vi "Read Landmarks From Text File.vi"(8 "error in":errorcluster, 10 "root VI's Path":path, 11 "File Name":string) -> (0 "error out":errorcluster, 3 "Landmarks":cluster{dbl, dbl}[](array[cluster]))   [LabVIEW 2009]
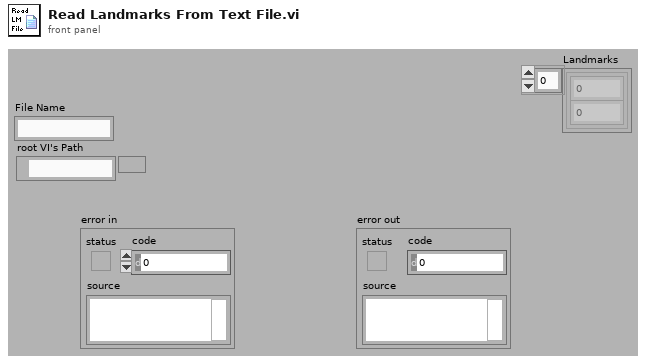
[diagram p1: front panel]
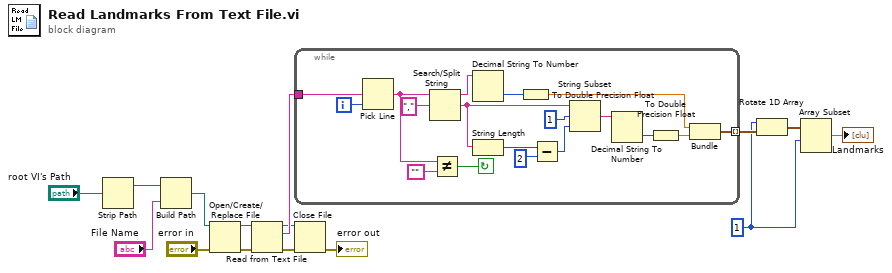
[diagram p0: block diagram]
diagram:
  w6 = 1 ("n")
  n1 = Strip Path(path="root VI's Path") -> (stripped path=w3:path)  [unwired: 1 out]
  n2 = Build Path(base path=w3, name or relative path="File Name") -> (appended path=w4:path)
  n3 = Open/Create/Replace File(file path (use dialog)=w4, error in="error in") -> (refnum out=w15:refnum<file>, error out=w14:errorcluster)  [unwired: 5 out]
  n4 = Read from Text File(file (use dialog)=w15, error in=w14) -> (refnum out=w12:refnum<file>, text=w13:string, error out=w11:errorcluster)  [unwired: 3 out]
  n5 = while {
    tunnel: w13 -> [w33]
    tunnel: [w23] -> w7 mode=indexing
    i -> [w32]
    stop <- w28 continue-if-true
    n6 = Pick Line(multi-line string=w33, line index=w32) -> (output string=w29:string)  [unwired: 1 out]
    n7 = Search/Split String(string=w29, search string/char (-)=",") -> (substring before match=w30:string, match + rest of string=w18:string)  [unwired: 2 out]
    n8 = Not Equal?(x=w29, y="") -> (x != y?=w28:bool)
    n9 = Decimal String To Number(string=w30) -> (number=w27:i32)  [unwired: 3 out]
    n10 = String Length(string=w18) -> (length=w21:i32)
    n11 = To Double Precision Float(number=w27) -> (double precision float=w24:dbl)
    n12 = Subtract(x=w21, y=2) -> (x-y=w19:i32)
    n13 = String Subset(string=w18, offset (0)=1, length (rest)=w19) -> (substring=w17:string)
    n14 = Decimal String To Number(string=w17) -> (number=w26:i32)  [unwired: 3 out]
    n15 = To Double Precision Float(number=w26) -> (double precision float=w25:dbl)
    n16 = Bundle(w24, w25) -> (w23:cluster{dbl, dbl})  [unwired: 1 out]
  }
  n17 = Close File(refnum=w12, error in=w11) -> (error out=→"error out":errorcluster)  [unwired: 1 out]
  n18 = Rotate 1D Array(1:w7, 2:w6) -> (0:w8:cluster{dbl, dbl}[])
  n19 = Array Subset(array=w8, index=w6) -> (→"Landmarks":cluster{dbl, dbl}[])  [unwired: 1 in]
